vi "calling_subvi.vi"() -> ()   [LabVIEW 2021]
doc: "本VI是为《我和LabVIEW》一书编写的示例。\n关于本书的介绍请参考网页：\nhttp://ruanqizhen.spaces.live.com/blog/cns!5852D4F797C53FB6!4310.entry"
panel:
  out "Waveform Graph":dbl[](graph)
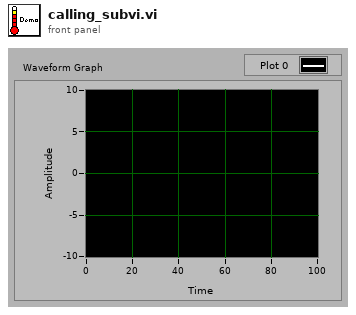
[diagram p1: front panel]
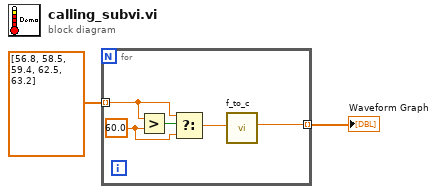
[diagram p0: block diagram]
diagram:
  n1 = for {
    tunnel: dbl[] [56.8, 58.5, 59.4, 62.5, 63.2] -> [w5] mode=indexing
    tunnel: [w7] -> w1 mode=indexing
    w4 = 60.0 ("y")
    n2 = Greater?(x=w5, y=w4) -> (0:w6:bool)
    n3 = Select(t=w5, s=w6, f=w4) -> (s? t:f=w3:dbl)
    n4 = call "f_to_c.vi"("Fahrenheit Temperature"=w3) -> ("Celsius Temperature"=w7:dbl)  [unwired: 8 in]
  }
  "Waveform Graph" <- w1
